vi "Local Dir to FTP Dir.vi"(7 "Root Path":path, 8 "error in (no error)":errorcluster, 10 "Path":path, 11 "FTPProtocol in":refnum<class "FTPProtocol.lvclass">) -> (0 "error out":errorcluster, 1 "parent folder in ftp":string, 2 "ftp path":string, 3 "FTPProtocol out":refnum<class "FTPProtocol.lvclass">)   [LabVIEW 2014, in "FileSync -- FTP.lvlib" / "FTPProtocol.lvclass"]
uses:
  FTPProtocol.lvclass
  FTPConfig/FTPConfig.lvclass
  FTPConfig/FTPConfig.lvclass/FTPConfig.ctl
  FTPConfig/Read config.vi
  <userlib>/_OpenG.lib/file/file.llb/Compare Two Paths - Scalar__ogtk.vi
  <userlib>/_OpenG.lib/array/array.llb/Filter 1D Array with Scalar (String)__ogtk.vi
  Base/ProtocolConfig/ProtocolConfig.lvclass
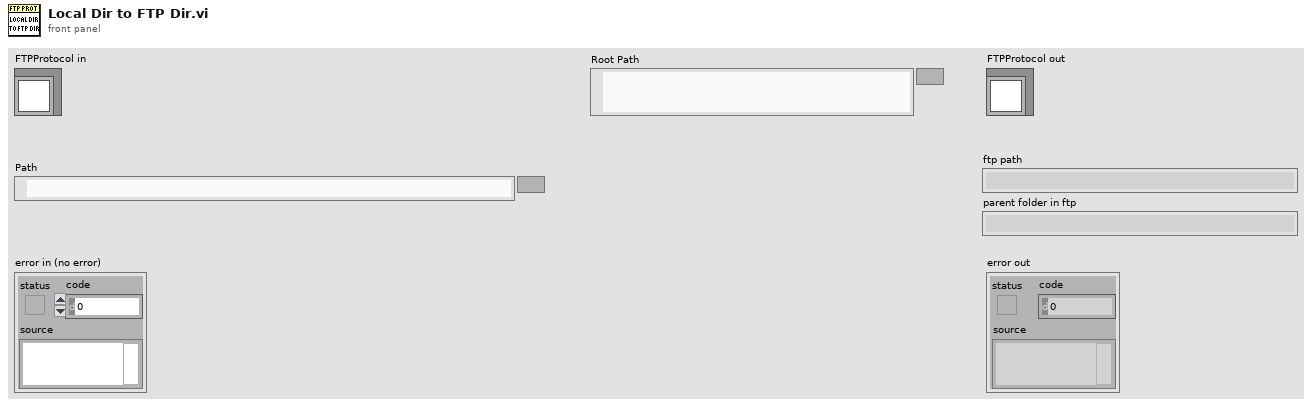
[diagram p1: front panel]
types:
  T1 = typedef "FileSync -- FTP.lvlib/FTPConfig.lvclass/Def-FTP Server Info.vi" = cluster{"address":string, "remote port":u16, "userName":string, "passWord":string, "RootDir":string}
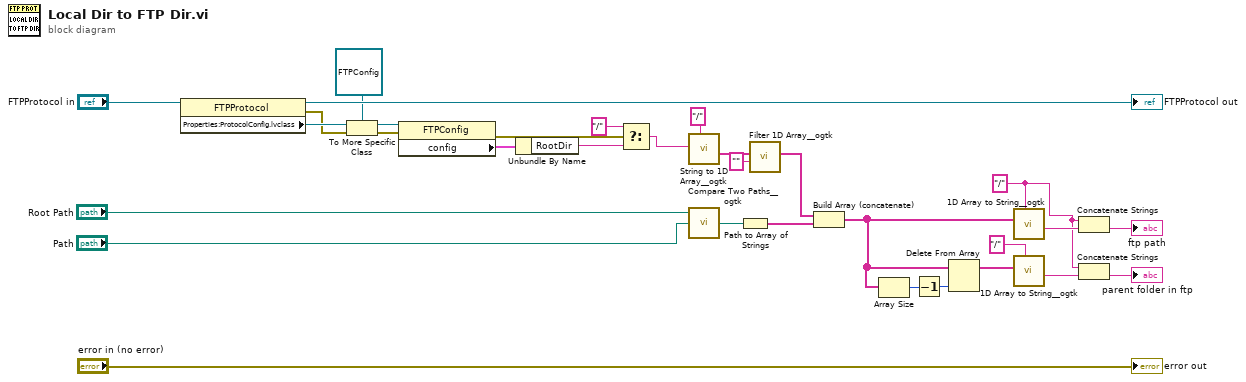
[diagram p0: block diagram]
diagram:
  w6 = "/" ("delimiter (Tab)")
  n1 = property class="FTPProtocol"(reference="FTPProtocol in") -> (reference out=→"FTPProtocol out":refnum<class "FTPProtocol.lvclass">, error out=w22:errorcluster, "Properties:ProtocolConfig.lvclass"=w25:refnum<class "ProtocolConfig.lvclass">)  [unwired: 1 in]
  n2 = To More Specific Class(target class=refnum<class "FTPConfig.lvclass"> refnum ("FTPConfig"), reference=w25, error in=w22) -> (specific class reference=w24:refnum<class "FTPConfig.lvclass">, error out=w21:errorcluster)
  n3 = property class="FTPConfig"(reference=w24, error in=w21) -> (error out=w4:errorcluster, "config"=w20:T1)  [unwired: 1 out]
  n4 = Unbundle By Name(w20) -> ("RootDir"=w3:string)
  n5 = Select(t="/" ("delimiter (Tab)"), s=w4, f=w3) -> (s? t:f=w2:string)
  n6 = call <userlib>:"String to 1D Array__ogtk.vi"("delimiter (Tab)"="/", "string"=w2) -> ("Array of Strings"=w18:string[])  [unwired: 9 in]
  n7 = call-poly <userlib>:"Compare Two Paths__ogtk.vi"("path2"="Path", "path1"="Root Path") -> ("relative path from 1 to 2"=w29:path)  [unwired: 1 in, 2 out]
  n8 = Path to Array of Strings(0:w29) -> (2:w5:string[])  [unwired: 1 out]
  n9 = call-poly <userlib>:"Filter 1D Array__ogtk.vi"("items to filter"="" ("delimiter (Tab)"), "array"=w18) -> ("filtered array"=w16:string[])  [unwired: 4 in, 1 out]
  n10 = Build Array (concatenate)(w16, w5) -> (w12:string[])
  n11 = Array Size(array=w12) -> (size(s)=w13:i32)
  n12 = Decrement(x=w13) -> (x-1=w14:i32)
  n13 = Delete From Array(array=w12, index=w14) -> (array with subset deleted=w10:string[])  [unwired: 1 in, 1 out]
  n14 = call <userlib>:"1D Array to String__ogtk.vi"("delimiter (Tab)"=w6, "Array of Strings"=w12) -> ("delimited string"=w15:string)  [unwired: 9 in]
  n15 = call <userlib>:"1D Array to String__ogtk.vi"("delimiter (Tab)"="/", "Array of Strings"=w10) -> ("delimited string"=w9:string)  [unwired: 9 in]
  n16 = Concatenate Strings(w6, w15) -> (→"ftp path":string)
  n17 = Concatenate Strings(w6, w9) -> (→"parent folder in ftp":string)
  "error out" <- "error in (no error)"
